vi "Total Consumption per day.vi"(11 "data":dbl[][](array[numeric])) -> (0 "mean":dbl format="%0.2f", 1 "XY Graph":cluster{"Y":dbl[], "Y":dbl[]}[](graph), 2 "total demand":dbl format="%0.2f", 3 "Total (kWh/day)":dbl[](array[numeric]), 4 "standard deviation":dbl format="%0.2f", 5 "variance":dbl format="%0.2f")   [LabVIEW 2018]
uses:
  <vilib>/Analysis/NI_AALBase.lvlib
panel:
  out "max index(es)":i32
  out "max value":dbl
  out "Waveform Graph":dbl[](graph)
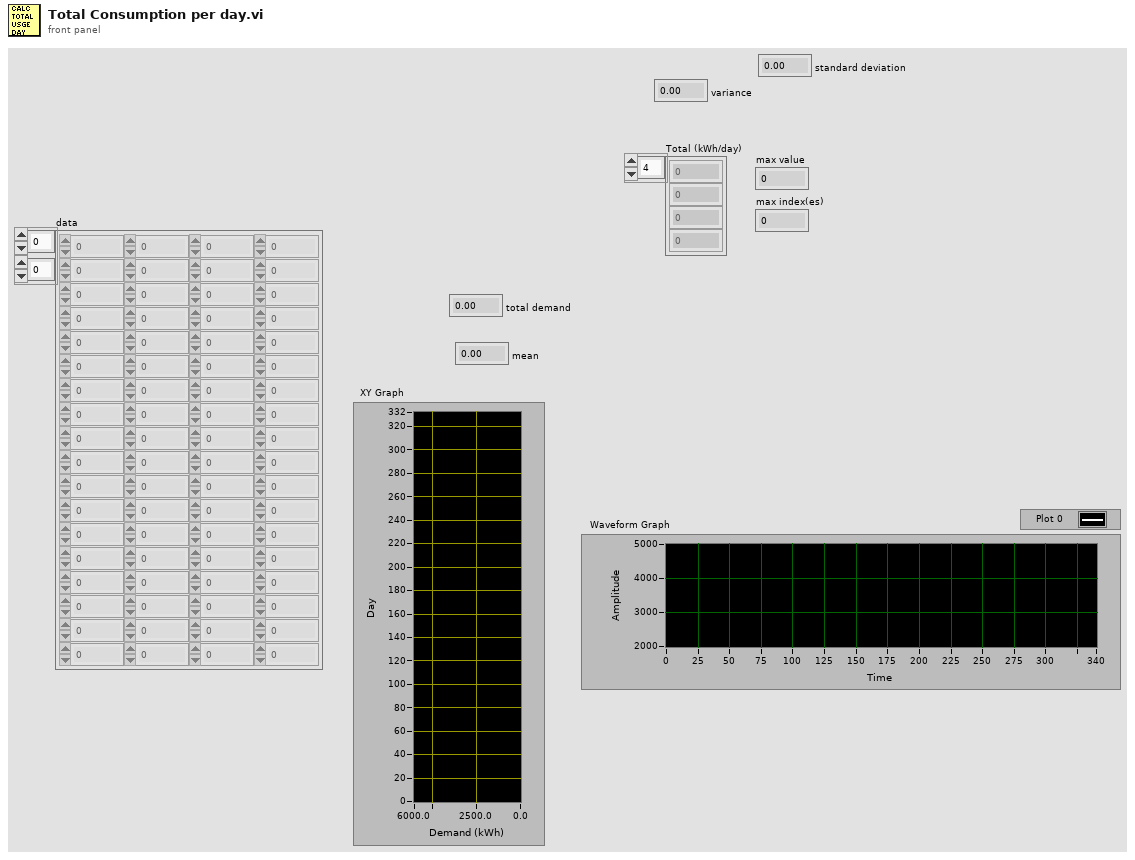
[diagram p1: front panel]
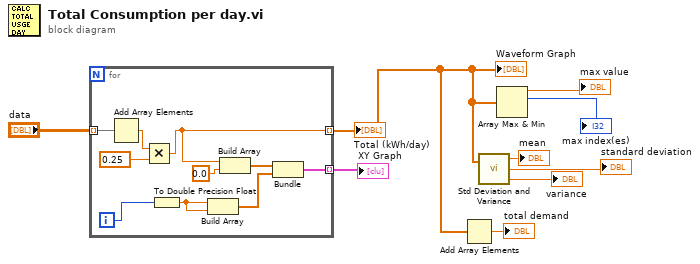
[diagram p0: block diagram]
diagram:
  n1 = for {
    tunnel: "data" -> [w19] mode=indexing
    tunnel: [w10] -> w3 mode=indexing
    tunnel: [w14] -> w9 mode=indexing
    i -> [w13]
    n2 = Add Array Elements(numeric array=w19) -> (sum=w11:dbl)
    n3 = Multiply(x=w11, y=0.25) -> (x*y=w10:dbl)
    n4 = To Double Precision Float(number=w13) -> (double precision float=w16:dbl)
    n5 = Build Array(w16, w16) -> (w18:dbl[])
    n6 = Build Array(w10, 0.0) -> (w17:dbl[])
    n7 = Bundle(w17, w18) -> (w14:cluster{dbl[], dbl[]})  [unwired: 1 in]
  }
  "Total (kWh/day)" <- w3
  "Waveform Graph" <- w3
  "XY Graph" <- w9
  n8 = Add Array Elements(numeric array=w3) -> (sum=→"total demand":dbl)
  n9 = call <vilib>:"Std Deviation and Variance.vi"("X"=w3) -> ("mean"=→"mean":dbl, "standard deviation"=→"standard deviation":dbl, "variance"=→"variance":dbl)  [unwired: 1 in]
  n10 = Array Max & Min(array=w3) -> (max value=→"max value":dbl, max index (indices)=→"max index(es)":i32)  [unwired: 2 out]
